vi "Run In UI.vi"(11 "LUnit Test Case in":refnum<class "LUnit Test Case.lvclass">) -> (3 "LUnit Test Case out":refnum<class "LUnit Test Case.lvclass">)   [LabVIEW 2020, in "LUnit Test Case.lvclass"]
uses:
  LUnit Test Case.lvclass
  LUnit Test Case.lvclass/LUnit Test Case.ctl
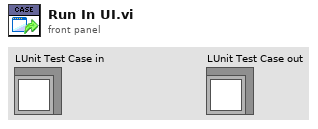
[diagram p1: front panel]
types:
  T1 = enum32{"Invalid", "Standard", "Closed", "Hidden", "Minimized", "Maximized"}
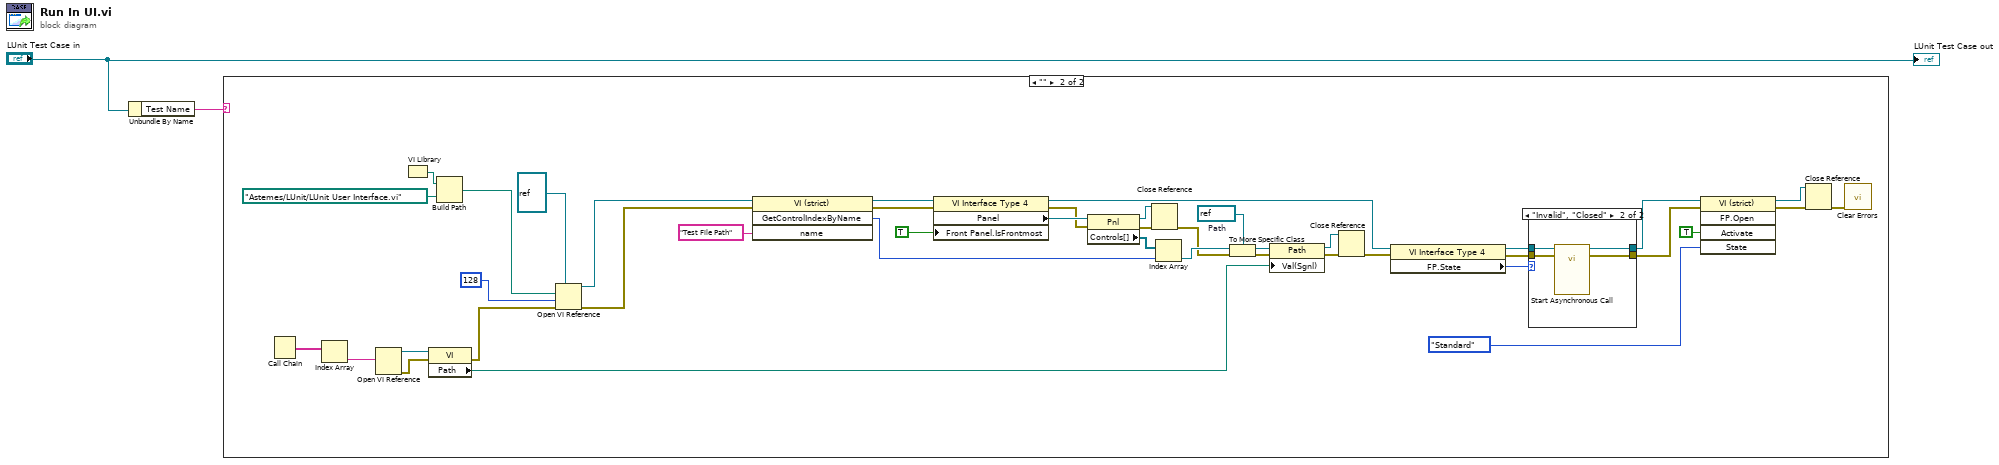
[diagram p0: block diagram]
diagram:
  n1 = Unbundle By Name("LUnit Test Case in") -> ("Test Name"=w1:string)
  n2 = case shown="\"\"" w1 {
    frame Default {
    }
    frame "" {
      w31 = refnum<vi> refnum  # Path
      n3 = Call Chain() -> (call chain=w3:string[])
      n4 = Index Array(array=w3) -> (element=w8:string)  [unwired: 1 in]
      n5 = Open VI Reference(vi path=w8) -> (vi reference=w7:refnum<vi>, error out=w4:errorcluster)  [unwired: 5 in]
      n6 = VI Library() -> (path=w37:path)
      n7 = property class="VI"(reference=w7, error in=w4) -> (error out=w5:errorcluster, "Path"=w6:path)  [unwired: 1 out]
      n8 = Build Path(base path=w37, name or relative path=path "Astemes/LUnit/LUnit User Interface.vi" ("Relative Path from 1 to 2")) -> (appended path=w42:path)
      n9 = Open VI Reference(type specifier VI Refnum (for type only)=refnum<vi> refnum, vi path=w42, options=128, error in (no error)=w5) -> (vi reference=w19:refnum<vi>, error out=w18:errorcluster)  [unwired: 2 in]
      n10 = invoke class="VI (strict)" method="GetControlIndexByName"(reference=w19, error in=w18, "name"="Test File Path" ("Control Name")) -> (reference out=w35:refnum<vi>, error out=w25:errorcluster, "GetControlIndexByName"=w32:i32)  [unwired: 1 in, 1 out]
      n11 = property class="VI Interface Type 4"(reference=w35, error in=w25, "Front Panel.IsFrontmost"=TRUE ("Front Panel Window:Is Frontmost")) -> (reference out=w12:refnum<vi>, error out=w26:errorcluster, "Panel"=w36:refnum<vi>)
      n12 = property class="Pnl"(reference=w36, error in=w26) -> (reference out=w22:refnum<vi>, error out=w27:errorcluster, "Controls[]"=w33:refnum<vi>[])
      n13 = Close Reference(reference=w22, error in (no error)=w27) -> (error out=w23:errorcluster)
      n14 = Index Array(array=w33, index=w32) -> (element=w29:refnum<vi>)
      n15 = To More Specific Class(target class=w31, reference=w29, error in=w23) -> (specific class reference=w30:refnum<vi>, error out=w28:errorcluster)
      n16 = property class="Path"(reference=w30, error in=w28, "Val(Sgnl)"=w6) -> (reference out=w21:refnum<vi>, error out=w24:errorcluster)
      n17 = Close Reference(reference=w21, error in (no error)=w24) -> (error out=w14:errorcluster)
      n18 = property class="VI Interface Type 4"(reference=w12, error in=w14) -> (reference out=w16:refnum<vi>, error out=w17:errorcluster, "FP.State"=w15:T1)
      n19 = case shown="\"Invalid\", \"Closed\"" w15 {
        tunnel: w17 -> [w46 w50]
        tunnel: w16 -> [w45 w49]
        tunnel: [w46 w47] -> w13
        tunnel: [w45 w48] -> w11
        frame Default {
        }
        frame "Invalid", "Closed" {
          n20 = call-by-ref "Start Asynchronous Call"(reference=w49, error in=w50) -> (reference out=w48:refnum<vi>, error out=w47:errorcluster)  [unwired: 12 in]
        }
      }
      n21 = invoke class="VI (strict)" method="FP.Open"(reference=w11, error in=w13, "Activate"=TRUE ("Activate?"), "State"=T1."Standard") -> (reference out=w41:refnum<vi>, error out=w40:errorcluster)  [unwired: 1 in, 3 out]
      n22 = Close Reference(reference=w41, error in (no error)=w40) -> (error out=w10:errorcluster)
      n23 = call <vilib>:"Clear Errors.vi"("error in (no error)"=w10) -> ()  [unwired: 5 in, 2 out]
    }
  }
  "LUnit Test Case out" <- "LUnit Test Case in"
